vi "module-04-xor-not.vi"() -> ()   [LabVIEW 2019]
panel:
  in  "Tab Control":enum32{"Execution", "Logic"}(tab)
  in  "XOR 1 -1":bool
  in  "XOR 1 - 2":bool
  in  "XOR 2-1":bool
  in  "XOR 2-2":bool
  in  "NOT 3":bool
  out "XOR 1 OUT":bool
  out "XOR 2 OUT":bool
  out "NOT 3 OUT":bool
  # "XOR  / NOT  GATE TEST"
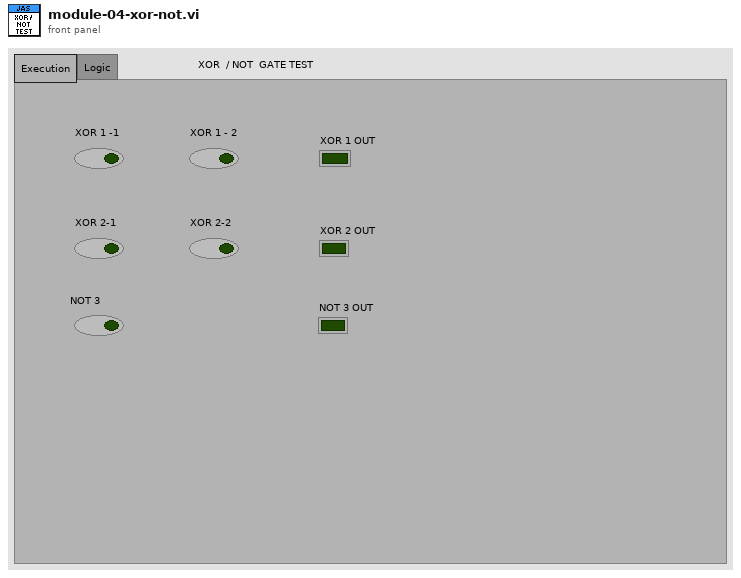
[diagram p1: front panel]
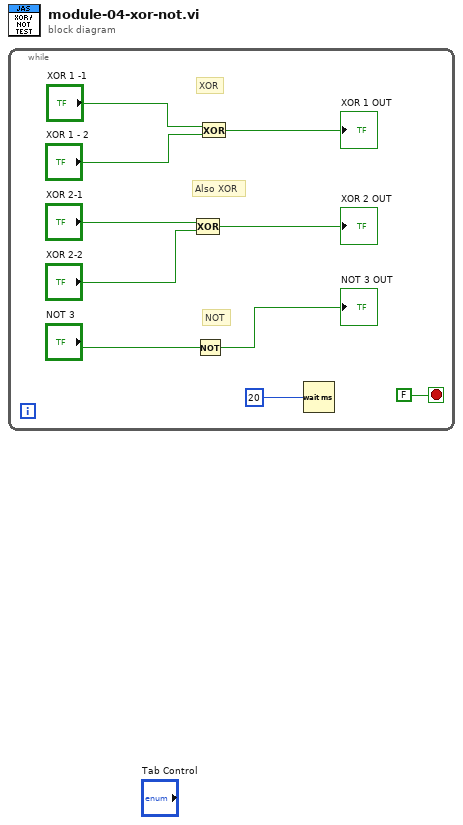
[diagram p0: block diagram]
diagram:
  n1 = while {
    stop <- FALSE stop-if-true
    # "NOT"
    # "Also XOR"
    # "XOR"
    n2 = Not(x="NOT 3") -> (.not. x?=→"NOT 3 OUT":bool)
    n3 = Compound Arithmetic op=XOR("XOR 2-1", "XOR 2-2") -> (→"XOR 2 OUT":bool)
    n4 = Exclusive Or(1:"XOR 1 - 2", 2:"XOR 1 -1") -> (0:→"XOR 1 OUT":bool)
    n5 = Wait (ms)(milliseconds to wait=u32 20) -> ()  [unwired: 1 out]
  }
